vi "Read.vi"(8 "error in":errorcluster, 10 "Channel":string, 11 "Buffer Lossless Bin in":refnum<class "Buffer Lossless Digital.lvclass">) -> (0 "error out":errorcluster, 1 "empty?":bool, 2 "Digital Waveform":digitalwaveform(waveform), 3 "Buffer Lossless Bin out":refnum<class "Buffer Lossless Digital.lvclass">)   [LabVIEW 2024, in "Buffer Lossless Digital.lvclass"]
uses:
  Buffer Lossless Digital.lvclass
  Buffer Lossless Digital.lvclass/Buffer Lossless Digital.ctl
  <vilib>/Waveform/DWDTOps.llb/DWDT Append Digital Samples.vi
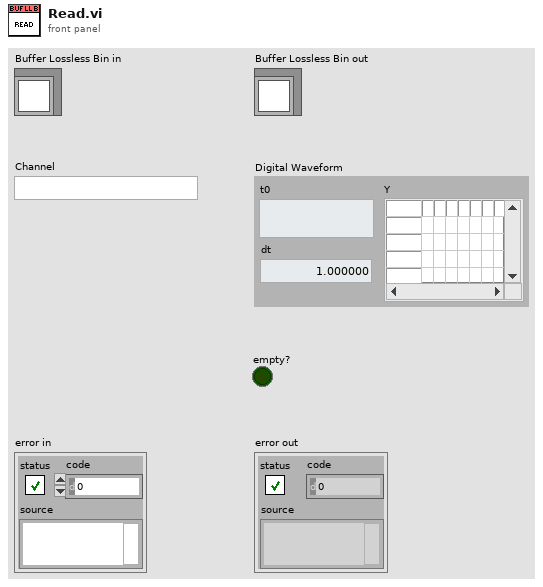
[diagram p1: front panel]
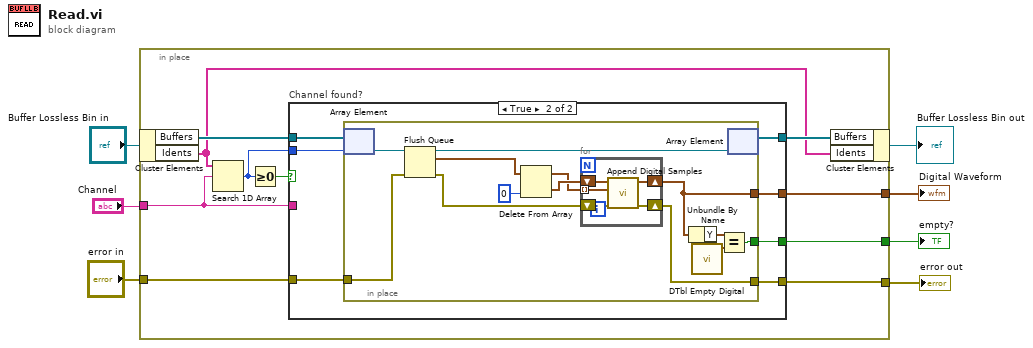
[diagram p0: block diagram]
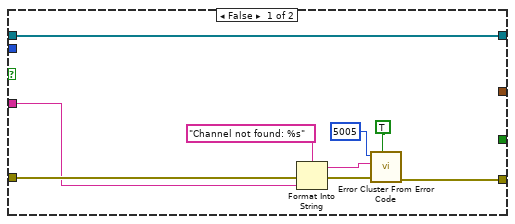
[diagram p2: hidden frame]
diagram:
  n1 = in-place {
    in-place-border: "Channel" -> [w8]
    in-place-border: "error in" -> [w17]
    in-place-border: [w16] -> w6
    in-place-border: [w15] -> w2
    in-place-border: [w9] -> w1
    n2 = in-place-cluster #1("Buffer Lossless Bin in") -> ("Buffers"=w12:refnum<queue>[], "Idents"=w10:string[])
    n3 = Search 1D Array(1D array=w10, element=w8) -> (index of element=w13:i32)  [unwired: 1 in]
    n4 = Greater Or Equal To 0?(x=w13) -> (x >= 0?=w14:bool)
    n5 = case "Channel found?" shown="True" w14 {
      tunnel: w17 -> [w21 w33]
      tunnel: [w20 w31] -> w16
      tunnel: [_ w32] -> w15
      tunnel: w13 -> [_ w29]
      tunnel: w12 -> [w19 w30]
      tunnel: [w19 w28] -> w11
      tunnel: [_ w27] -> w9
      tunnel: w8 -> [w18 _]
      frame False {
        n6 = Format Into String(format string="Channel not found: %s", error in=w21, w18) -> (resulting string=w22:string, error out=w24:errorcluster)  [unwired: 1 in]
        n7 = call <vilib>:"Error Cluster From Error Code.vi"("show call chain? (False)"=TRUE, "error in (no error)"=w24, "error message (\"\")"=w22, "error code (0)"=5005) -> ("error out"=w20:errorcluster)  [unwired: 5 in]
      }
      frame True {
        n8 = in-place {
          in-place-border: w33 -> [w46]
          in-place-border: [w41] -> w32
          in-place-border: [w42] -> w31
          in-place-border: [w38] -> w27
          n9 = in-place-array #2(w30, w29) -> (w45:refnum<queue>)
          n10 = Flush Queue(queue=w45, error in (no error)=w46) -> (queue out=w44:refnum<queue>, remaining elements=w37:digitalwaveform[], error out=w43:errorcluster)
          n11 = Delete From Array(array=w37, index=0) -> (deleted portion=w35:digitalwaveform, array with subset deleted=w34:digitalwaveform[])  [unwired: 1 in]
          n12 = for {
            tunnel: w34 -> [w50] mode=indexing
            shift-right: [w47] -> w41
            shift-left: w35 -> [w51]
            shift-right: [w48] -> w42
            shift-left: w43 -> [w49]
            n13 = call-poly <vilib>:"Append Digital Samples.vi"("error in (no error)"=w49, "digital waveform B"=w50, "digital waveform A"=w51) -> ("error out"=w48:errorcluster, "digital waveform out"=w47:digitalwaveform)  [unwired: 7 in]
          }
          n14 = Unbundle By Name(w41) -> ("Y"=w40:digitaldata)
          n15 = call <vilib>:"DTbl Empty Digital.vi"() -> ("digital data"=w39:digitaldata)  [unwired: 5 in]
          n16 = Equal?(x=w40, y=w39) -> (x = y?=w38:bool)
          n17 = in-place-array #2(w44) -> (w28:refnum<queue>[])  [unwired: 1 out]
        }
      }
    }
    n18 = in-place-cluster #1("Buffers"=w11, "Idents"=w10) -> (→"Buffer Lossless Bin out":refnum<class "Buffer Lossless Digital.lvclass">)
  }
  "error out" <- w6
  "Digital Waveform" <- w2
  "empty?" <- w1
